vi "Attacker Stop.vi"(6 "atacando contra?":bool, 8 "IA State Input 2":T1, 9 "balls":T4[](array[typedef]), 10 "Field Size in":T5, 11 "Robot in":T2) -> (3 "Robot out":T2)   [LabVIEW 2016]
uses:
  Core/Field Size.ctl
  Core/AI Robot.ctl
  Functions Enum.ctl
  Core/AI Ball.ctl
  Core/AI Input.ctl
  Core/AI Judge.ctl
  Command Enum.ctl
  <vilib>/Analysis/_algsub.llb/Real Vector Norm.vi
  <vilib>/Analysis/NI_AALPro.lvlib
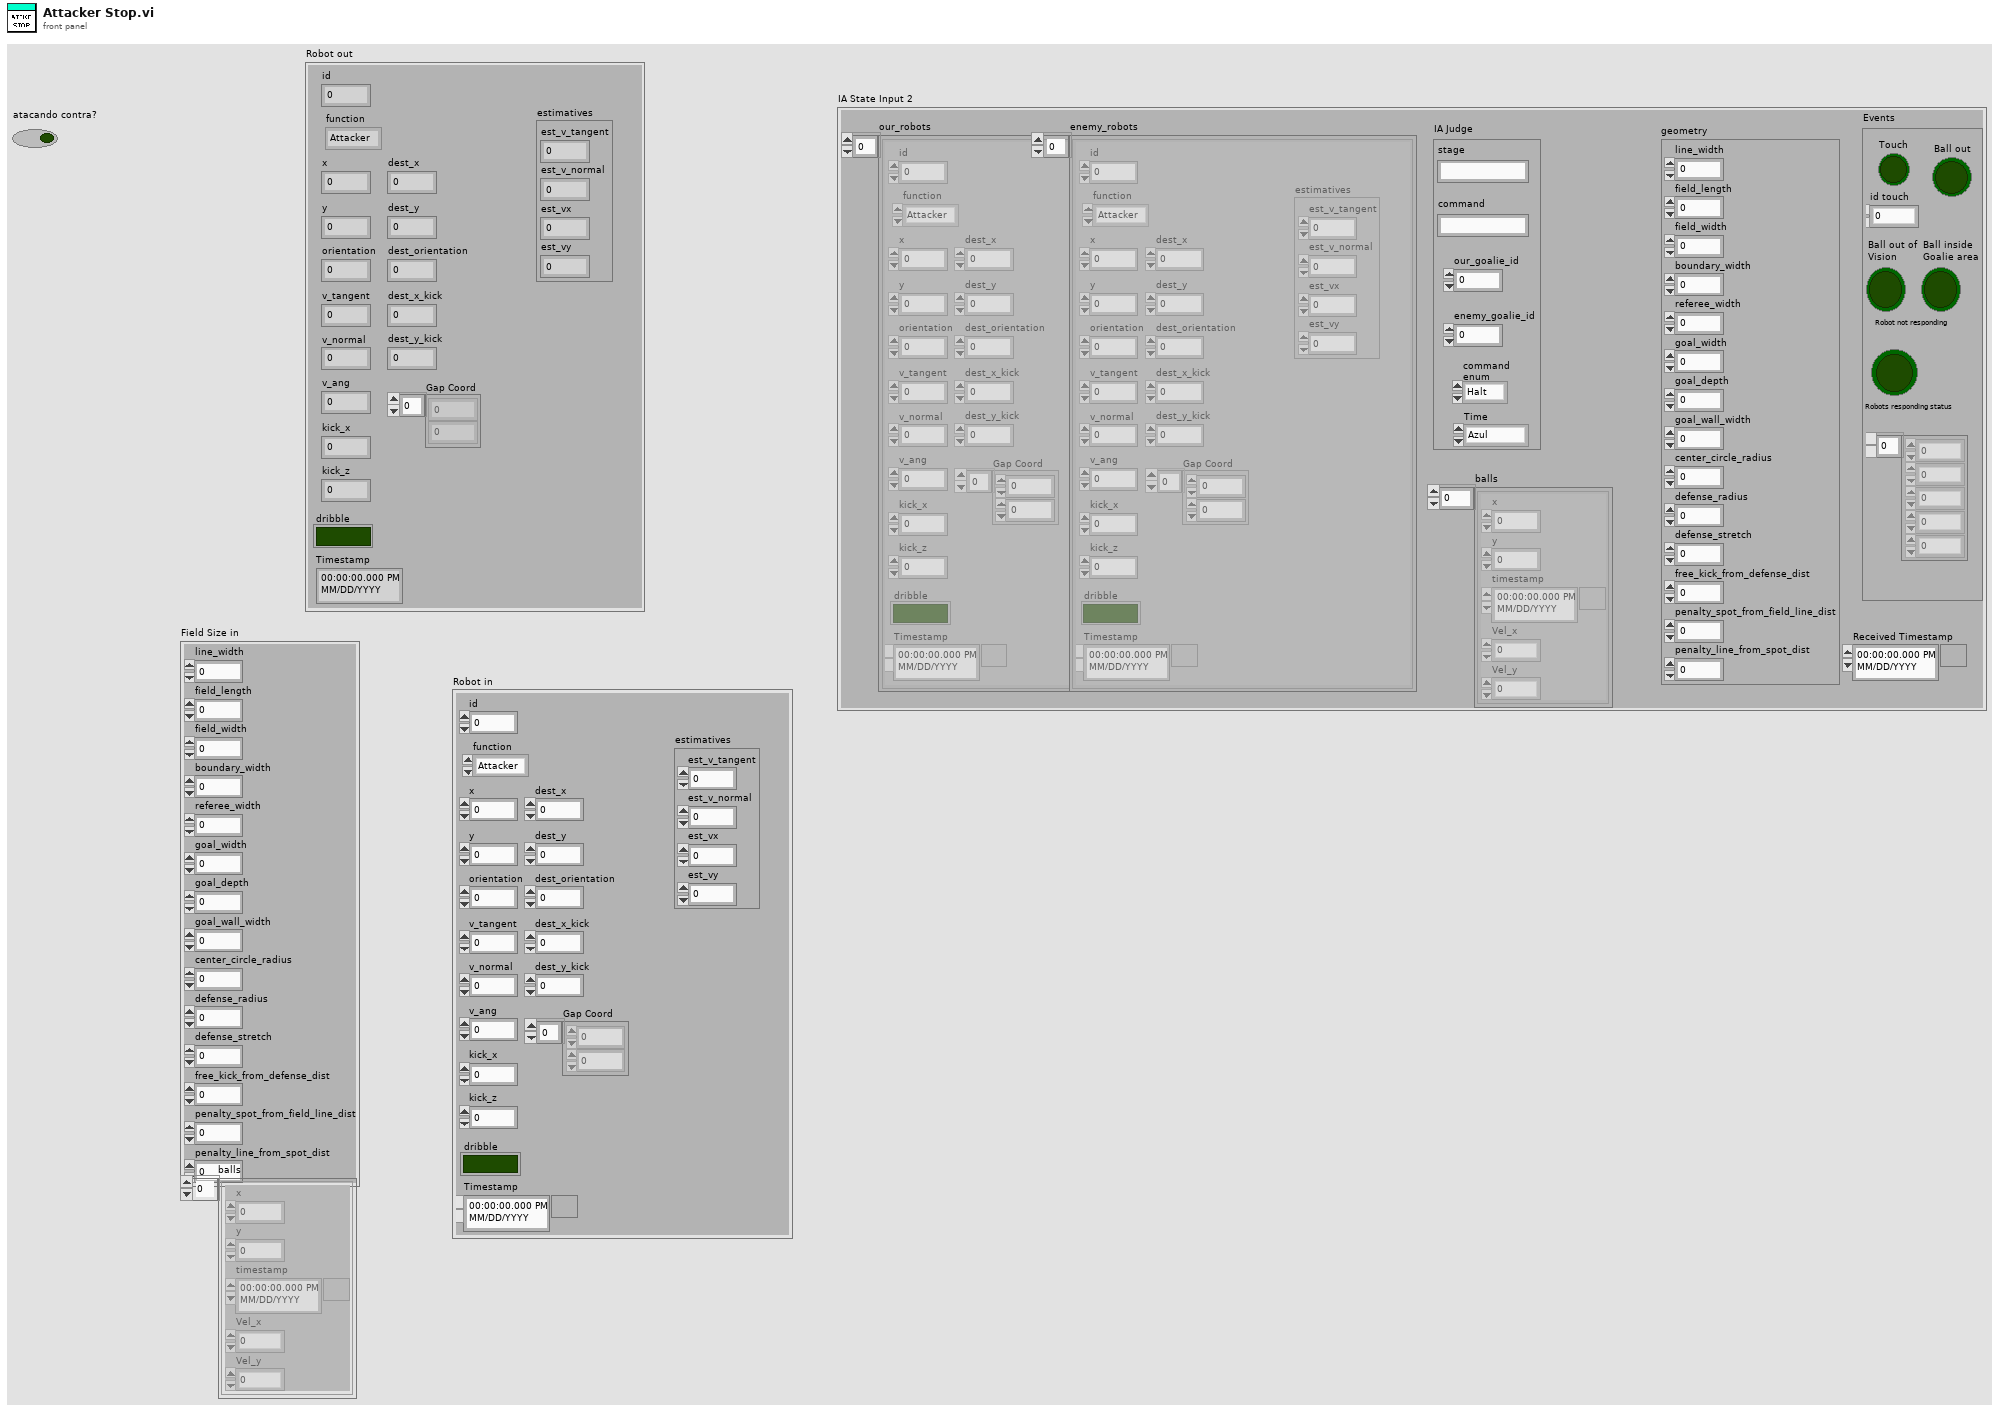
[diagram p1: front panel]
types:
  T1 = typedef "AI Input.ctl" = cluster{"our_robots":T2[], "enemy_robots":T2[], "balls":T4[], "geometry":T5, "IA Judge":T6, "Received Timestamp":timestamp, "Events":cluster{"Touch":bool, "Ball out":bool, "id touch":dbl, "Ball out of \nVision":bool, "Ball inside \nGoalie area":bool, "Robot not responding":bool, "Robots responding status":dbl[]}}
  T2 = typedef "AI Robot.ctl" = cluster{"id":u32, "function":T3, "x":dbl, "y":dbl, "orientation":dbl, "v_tangent":dbl, "v_normal":dbl, "v_ang":dbl, "kick_x":dbl, "kick_z":dbl, "dribble":bool, "Timestamp":timestamp, "dest_x":dbl, "dest_y":dbl, "dest_orientation":dbl, "estimatives":cluster{"est_v_tangent":dbl, "est_v_normal":dbl, "est_vx":dbl, "est_vy":dbl}, "dest_x_kick":dbl, "dest_y_kick":dbl, "Gap Coord":dbl[]}
  T3 = typedef "Functions Enum.ctl" = enum16{"Attacker", "Goalie", "Defender", "Striker", "Goto 0", "Dummy", "Kicker", "ZigZag"}
  T4 = typedef "AI Ball.ctl" = cluster{"x":dbl, "y":dbl, "timestamp":timestamp, "Vel_x":dbl, "Vel_y":dbl}
  T5 = typedef "Field Size.ctl" = cluster{"line_width":u32, "field_length":u32, "field_width":u32, "boundary_width":u32, "referee_width":u32, "goal_width":u32, "goal_depth":u32, "goal_wall_width":u32, "center_circle_radius":u32, "defense_radius":u32, "defense_stretch":u32, "free_kick_from_defense_dist":u32, "penalty_spot_from_field_line_dist":u32, "penalty_line_from_spot_dist":u32}
  T6 = typedef "AI Judge.ctl" = cluster{"stage":string, "command":string, "our_goalie_id":dbl, "enemy_goalie_id":dbl, "command\nenum":T7, "Time":enum16{"Azul", "Amarelo"}}
  T7 = typedef "Command Enum.ctl" = enum16{"Halt", "Stop", "Force Start", "PKA Normal Start", "Prepare Kickoff Ally", "PKE Normal Start", "Prepare Kickoff Enemy", "Prepare Penalty Ally", "PPA Normal Start", "Prepare Penalty Enemy", "PPE Normal Start", "Direct Free Enemy", "Direct Free Ally", "Indirect Free Enemy", "Indirect Free Ally", "Timeout Enemy", "Timeout Ally", "Goal Enemy", "Goal Ally", "Ball Placement Enemy", "Ball Placement Ally", "None"}
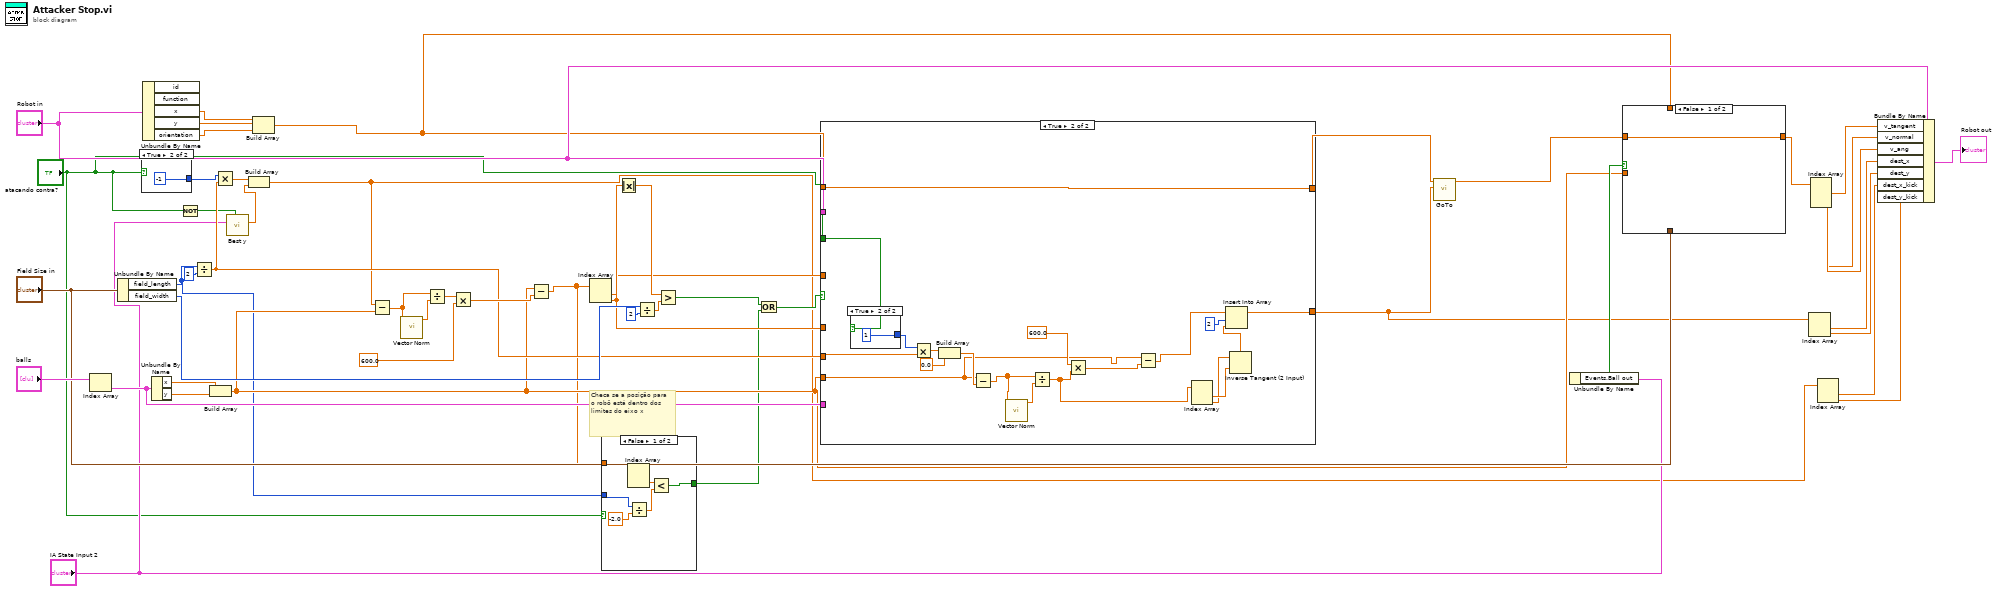
[diagram p0: block diagram]
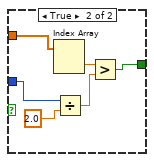
[diagram p2: hidden frame]
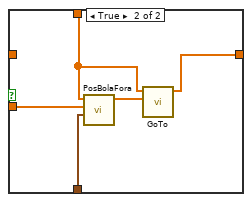
[diagram p3: hidden frame]
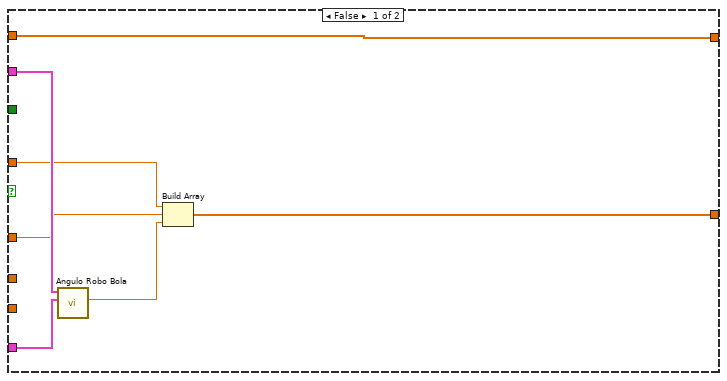
[diagram p4: hidden frame]
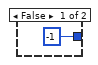
[diagram p5: hidden frame]
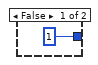
[diagram p6: hidden frame]
diagram:
  # "Checa se a posição para o robõ está dentro dos limites do eixo x"
  n1 = Index Array(array="balls") -> (element=w36:T4)  [unwired: 1 in]
  n2 = Unbundle By Name("Field Size in") -> ("field_length"=w13:u32, "field_width"=w38:u32)
  n3 = case shown="True" "atacando contra?" {
    tunnel: [1 -1] -> w47
    frame False {
    }
    frame True {
    }
  }
  n4 = Unbundle By Name("Robot in") -> ("x"=w33:dbl, "y"=w32:dbl, "orientation"=w31:dbl)  [unwired: 2 out]
  n5 = Unbundle By Name(w36) -> ("x"=w46:dbl, "y"=w45:dbl)
  n6 = Not(x="atacando contra?") -> (.not. x?=w5:bool)
  n7 = Divide(x=w13, y=u32 2) -> (x/y=w16:dbl)
  n8 = Build Array(w46, w45) -> (w15:dbl[])
  n9 = Multiply(x=w47, y=w16) -> (x*y=w44:dbl)
  n10 = call "Best y.vi"("inimigos"=w5, "IA State"="IA State Input 2") -> ("Best y"=w6:dbl)  [unwired: 6 in, 3 out]
  n11 = Build Array(w44, w6) -> (w3:dbl[])
  n12 = Build Array(w33, w32, w31) -> (w22:dbl[])
  n13 = Subtract(x=w3, y=w15) -> (x-y=w43:dbl[])
  n14 = call-poly <vilib>:"Vector Norm.vi"("Input Vector"=w43) -> ("norm"=w42:dbl)  [unwired: 9 in, 1 out]
  n15 = Divide(x=w43, y=w42) -> (x/y=w41:dbl[])
  n16 = Multiply(x=w41, y=600.0) -> (x*y=w19:dbl[])
  n17 = Subtract(x=w15, y=w19) -> (x-y=w14:dbl[])
  n18 = Index Array(array=w14) -> (element #1=w34:dbl, element #2=w35:dbl)  [unwired: 2 in]
  n19 = case shown="False" "atacando contra?" {
    tunnel: w13 -> [w55 w61]
    tunnel: [w54 w58] -> w8
    tunnel: w14 -> [w53 w62]
    frame False {
      n20 = Index Array(array=w53) -> (element #1=w57:dbl)  [unwired: 2 in, 1 out]
      n21 = Divide(x=w55, y=-2.0) -> (x/y=w56:dbl)
      n22 = Less?(x=w57, y=w56) -> (x < y?=w54:bool)
    }
    frame True {
      n23 = Index Array(array=w62) -> (element #1=w60:dbl)  [unwired: 2 in, 1 out]
      n24 = Divide(x=w61, y=2.0) -> (x/y=w59:dbl)
      n25 = Greater?(x=w60, y=w59) -> (0:w58:bool)
    }
  }
  n26 = Absolute Value(x=w35) -> (abs(x)=w40:dbl)
  n27 = Divide(x=w38, y=u32 2) -> (x/y=w37:dbl)
  n28 = Greater?(x=w40, y=w37) -> (0:w9:bool)
  n29 = Or(x=w9, y=w8) -> (x .or. y?=w10:bool)
  n30 = case shown="True" w10 {
    tunnel: w36 -> [w70 _]
    tunnel: "Robot in" -> [w69 _]
    tunnel: w35 -> [w67 _]
    tunnel: w34 -> [w66 _]
    tunnel: w22 -> [w65 w76]
    tunnel: w15 -> [_ w72]
    tunnel: "atacando contra?" -> [_ w83]
    tunnel: w16 -> [_ w88]
    tunnel: [w65 w76] -> w12
    tunnel: [w64 w75] -> w11
    frame False {
      n31 = call "Angulo Robo Bola.vi"("Ball"=w70, "Robot"=w69) -> ("Angulo"=w68:dbl)  [unwired: 9 in]
      n32 = Build Array(w66, w67, w68) -> (w64:dbl[])
    }
    frame True {
      n33 = case shown="True" w83 {
        tunnel: [-1 1] -> w89
        frame False {
        }
        frame True {
        }
      }
      n34 = Multiply(x=w89, y=w88) -> (x*y=w87:dbl)
      n35 = Build Array(w87, 0.0 ("element")) -> (w82:dbl[])
      n36 = Subtract(x=w72, y=w82) -> (x-y=w84:dbl[])
      n37 = call-poly <vilib>:"Vector Norm.vi"("Input Vector"=w84) -> ("norm"=w85:dbl)  [unwired: 9 in, 1 out]
      n38 = Divide(x=w84, y=w85) -> (x/y=w77:dbl[])
      n39 = Multiply(x=600.0, y=w77) -> (x*y=w73:dbl[])
      n40 = Subtract(x=w72, y=w73) -> (x-y=w71:dbl[])
      n41 = Index Array(array=w77) -> (element #1=w79:dbl, element #2=w78:dbl)  [unwired: 2 in]
      n42 = Inverse Tangent (2 Input)(1:w79, 2:w78) -> (0:w80:dbl)
      n43 = Insert Into Array(array=w71, index=2, new element=w80) -> (w75:dbl[])
    }
  }
  n44 = call "GoTo.vi"("Target"=w11, "Position"=w12) -> ("Output\nVelocity"=w21:dbl[])  [unwired: 8 in, 1 out]
  n45 = Unbundle By Name("IA State Input 2") -> ("Events.Ball out"=w30:bool)
  n46 = case shown="False" w30 {
    tunnel: w21 -> [w92 _]
    tunnel: [w92 w93] -> w24
    tunnel: "Field Size in" -> [_ w97]
    tunnel: w22 -> [_ w94]
    tunnel: w15 -> [_ w96]
    frame False {
    }
    frame True {
      n47 = call "PosBolaFora.vi"("Field Size in"=w97, "Position da bola"=w96, "Position do robot"=w94) -> ("Target"=w95:dbl[])  [unwired: 8 in]
      n48 = call "GoTo.vi"("Target"=w95, "Position"=w94) -> ("Output\nVelocity"=w93:dbl[])  [unwired: 8 in, 1 out]
    }
  }
  n49 = Index Array(array=w11) -> (element #1=w18:dbl, element #2=w17:dbl)  [unwired: 2 in]
  n50 = Index Array(array=w24) -> (element #1=w27:dbl, element #2=w28:dbl, element #3=w29:dbl)  [unwired: 3 in]
  n51 = Index Array(array=w3) -> (element #1=w2:dbl, element #2=w1:dbl)  [unwired: 2 in]
  n52 = Bundle By Name(cluster="Robot in", "v_tangent"=w27, "v_normal"=w28, "v_ang"=w29, "dest_x"=w18, "dest_y"=w17, "dest_x_kick"=w2, "dest_y_kick"=w1) -> (→"Robot out":T2)
